vi "DiffDrivePoseEst2_UpdateWithTime.vi"(6 "CurrentTimeSeconds":dbl=-1.0, 8 "RightDistance":dbl, 9 "LeftDistance":dbl, 10 "GyroAngle":T3={"VALUE"=0.0, "COS"=1.0, "SIN"=0.0} {"SIN" format="%13.4f"; "COS" format="%13.4f"; "VALUE" format="%13.4f"}, 11 "in DiffDrivePoseEst2":T4={"M_Vision_K"=[], "m_nominal_dT"=0.0, "m_PrevTime_Sec"=0.0, "Pose_Buffer"={"TimeStamps"=[], "DataArray"=[], "Min_TimeStamp"=0.0, "Max_TimeStamp"=0.0, "ItemCount"=0, "MaxBufferTime"=0.0}, "Diff_Drive_Kinematics"={"TrackWidth_Meters"=0.0}, "Diff_Drive_Odom_2"={"M_POSE_Meters"={"TRANSLATION"={"X"=0.0, "Y"=0.0}, "ROTATION"={"VALUE"=0.0, "COS"=1.0, "SIN"=0.0}}, "M_GyroOffset"={"VALUE"=0.0, "COS"=1.0, "SIN"=0.0}, "M_PrevAngle"={"VALUE"=0.0, "COS"=1.0, "SIN"=0.0}, "M_PrevLeftDist_M"=0.0, "M_PrevRightDist_M"=0.0, "M_InitLeftDist_M"=0.0, "M_InitRightDist_M"=0.0}, "M_Q"=[[0.0], [0.0], [0.0]]} {"Diff_Drive_Odom_2"."M_PrevAngle"."SIN" format="%13.4f"; "Diff_Drive_Odom_2"."M_PrevAngle"."COS" format="%13.4f"; "Diff_Drive_Odom_2"."M_PrevAngle"."VALUE" format="%13.4f"; "Diff_Drive_Odom_2"."M_GyroOffset"."SIN" format="%13.4f"; "Diff_Drive_Odom_2"."M_GyroOffset"."COS" format="%13.4f"; "Diff_Drive_Odom_2"."M_GyroOffset"."VALUE" format="%13.4f"; "Diff_Drive_Odom_2"."M_POSE_Meters"."ROTATION"."SIN" format="%13.4f"; "Diff_Drive_Odom_2"."M_POSE_Meters"."ROTATION"."COS" format="%13.4f"; "Diff_Drive_Odom_2"."M_POSE_Meters"."ROTATION"."VALUE" format="%13.4f"; "Diff_Drive_Odom_2"."M_POSE_Meters"."TRANSLATION"."Y" format="%14.3f"; "Diff_Drive_Odom_2"."M_POSE_Meters"."TRANSLATION"."X" format="%14.3f"; "Diff_Drive_Kinematics"."TrackWidth_Meters" format="%20.4f"}) -> (0 "Error":bool, 2 "Estimated Pose":T1 {"ROTATION"."SIN" format="%13.4f"; "ROTATION"."COS" format="%13.4f"; "ROTATION"."VALUE" format="%13.4f"; "TRANSLATION"."Y" format="%14.3f"; "TRANSLATION"."X" format="%14.3f"}, 3 "Out DiffDrivePoseEst2":T4={"M_Vision_K"=[], "m_nominal_dT"=0.0, "m_PrevTime_Sec"=0.0, "Pose_Buffer"={"TimeStamps"=[], "DataArray"=[], "Min_TimeStamp"=0.0, "Max_TimeStamp"=0.0, "ItemCount"=0, "MaxBufferTime"=0.0}, "Diff_Drive_Kinematics"={"TrackWidth_Meters"=0.0}, "Diff_Drive_Odom_2"={"M_POSE_Meters"={"TRANSLATION"={"X"=0.0, "Y"=0.0}, "ROTATION"={"VALUE"=0.0, "COS"=1.0, "SIN"=0.0}}, "M_GyroOffset"={"VALUE"=0.0, "COS"=1.0, "SIN"=0.0}, "M_PrevAngle"={"VALUE"=0.0, "COS"=1.0, "SIN"=0.0}, "M_PrevLeftDist_M"=0.0, "M_PrevRightDist_M"=0.0, "M_InitLeftDist_M"=0.0, "M_InitRightDist_M"=0.0}, "M_Q"=[[0.0], [0.0], [0.0]]} {"Diff_Drive_Odom_2"."M_PrevAngle"."SIN" format="%13.4f"; "Diff_Drive_Odom_2"."M_PrevAngle"."COS" format="%13.4f"; "Diff_Drive_Odom_2"."M_PrevAngle"."VALUE" format="%13.4f"; "Diff_Drive_Odom_2"."M_GyroOffset"."SIN" format="%13.4f"; "Diff_Drive_Odom_2"."M_GyroOffset"."COS" format="%13.4f"; "Diff_Drive_Odom_2"."M_GyroOffset"."VALUE" format="%13.4f"; "Diff_Drive_Odom_2"."M_POSE_Meters"."ROTATION"."SIN" format="%13.4f"; "Diff_Drive_Odom_2"."M_POSE_Meters"."ROTATION"."COS" format="%13.4f"; "Diff_Drive_Odom_2"."M_POSE_Meters"."ROTATION"."VALUE" format="%13.4f"; "Diff_Drive_Odom_2"."M_POSE_Meters"."TRANSLATION"."Y" format="%14.3f"; "Diff_Drive_Odom_2"."M_POSE_Meters"."TRANSLATION"."X" format="%14.3f"; "Diff_Drive_Kinematics"."TrackWidth_Meters" format="%20.4f"})   [LabVIEW 2019, in "Trajectory_Library.lvlib"]
doc: "Updates the the Unscented Kalman Filter using only wheel encoder information. Note that this should be called every loop.\n\nInputs:\n - LeftSpeed -- Left wheel speed (meters/sec)\n - RightSpeed -- Right wheel speed (meters/sec)\n - inDiffDrivePoseEst -- system data cluster\n - gyroAngle -- The current gyro angle. (radians)\n - currentTime -- Time at which this method was called, in seconds.\n - distanceLeftMeters -- The total distance travelled by the left wheel in meters. This can be the encoder reading.\n - distanceRightMeters -- The total distance travelled by the right wheel in meters. This can be the encoder reading.\n\nOutputs:\n - outDiffDrivePoseEst -- system data cluster\n - EstimatedPose -- The estimated pose of the robot in meters."
uses:
  Trajectory_Library.lvlib
  <vilib>/Analysis/Matrix/Datatypes/RealMatrix.ctl
  <vilib>/Analysis/Matrix/NI_Matrix.lvlib
  TypeDef/ROTATION2D.ctl
  TypeDef/TRANSLATION2D.ctl
  TypeDef/POSE2D.ctl
  TypeDef/TIME_INTERPOLATABLE_VARIANT.ctl
  TypeDef/DIFF_DRIVE_KINEMATICS.ctl
  TypeDef/DIFF_DRIVE_ODOM2.ctl
  TypeDef/DIFF_DRIVE_POSE_EST2.ctl
panel:
  # "<3, 1>"
  # "<3, 3>"
  # "<3, 1>"
  # "<3, 3>"
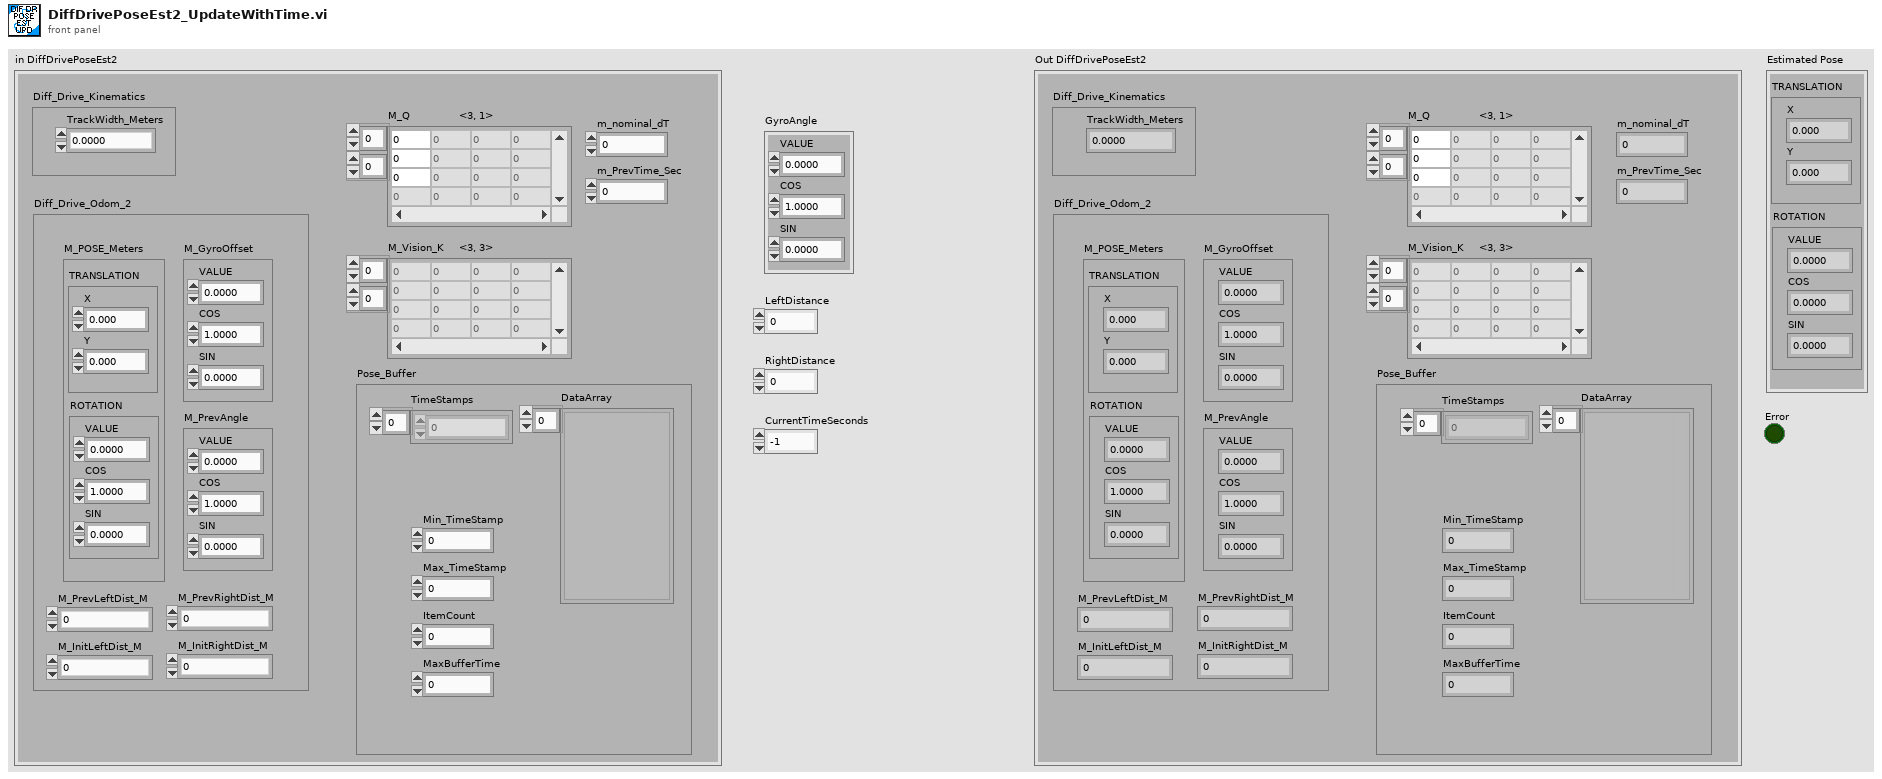
[diagram p1: front panel]
types:
  T1 = typedef "Trajectory_Library.lvlib/POSE2D.ctl" = cluster{"TRANSLATION":T2, "ROTATION":T3}
  T2 = typedef "Trajectory_Library.lvlib/TRANSLATION2D.ctl" = cluster{"X":dbl, "Y":dbl}
  T3 = typedef "Trajectory_Library.lvlib/ROTATION2D.ctl" = cluster{"VALUE":dbl, "COS":dbl, "SIN":dbl}
  T4 = typedef "Trajectory_Library.lvlib/DIFF_DRIVE_POSE_EST2.ctl" = cluster{"M_Vision_K":T5, "m_nominal_dT":dbl, "m_PrevTime_Sec":dbl, "Pose_Buffer":T6, "Diff_Drive_Kinematics":T7, "Diff_Drive_Odom_2":T8, "M_Q":T5}
  T5 = typedef "NI_Matrix.lvlib/RealMatrix.ctl" = dbl[][]
  T6 = typedef "Trajectory_Library.lvlib/TIME_INTERPOLATABLE_VARIANT.ctl" = cluster{"TimeStamps":dbl[], "DataArray":variant[], "Min_TimeStamp":dbl, "Max_TimeStamp":dbl, "ItemCount":i32, "MaxBufferTime":dbl}
  T7 = typedef "Trajectory_Library.lvlib/DIFF_DRIVE_KINEMATICS.ctl" = cluster{"TrackWidth_Meters":dbl}
  T8 = typedef "Trajectory_Library.lvlib/DIFF_DRIVE_ODOM2.ctl" = cluster{"M_POSE_Meters":T1, "M_GyroOffset":T3, "M_PrevAngle":T3, "M_PrevLeftDist_M":dbl, "M_PrevRightDist_M":dbl, "M_InitLeftDist_M":dbl, "M_InitRightDist_M":dbl}
  T9 = typedef "Trajectory_Library.lvlib/DIFF_DRIVE_POSE_EST2_INTERP_RECORD.ctl" = cluster{"PoseMeters":T1, "GyroAngle":T3, "LeftMeters":dbl, "RightMeters":dbl}
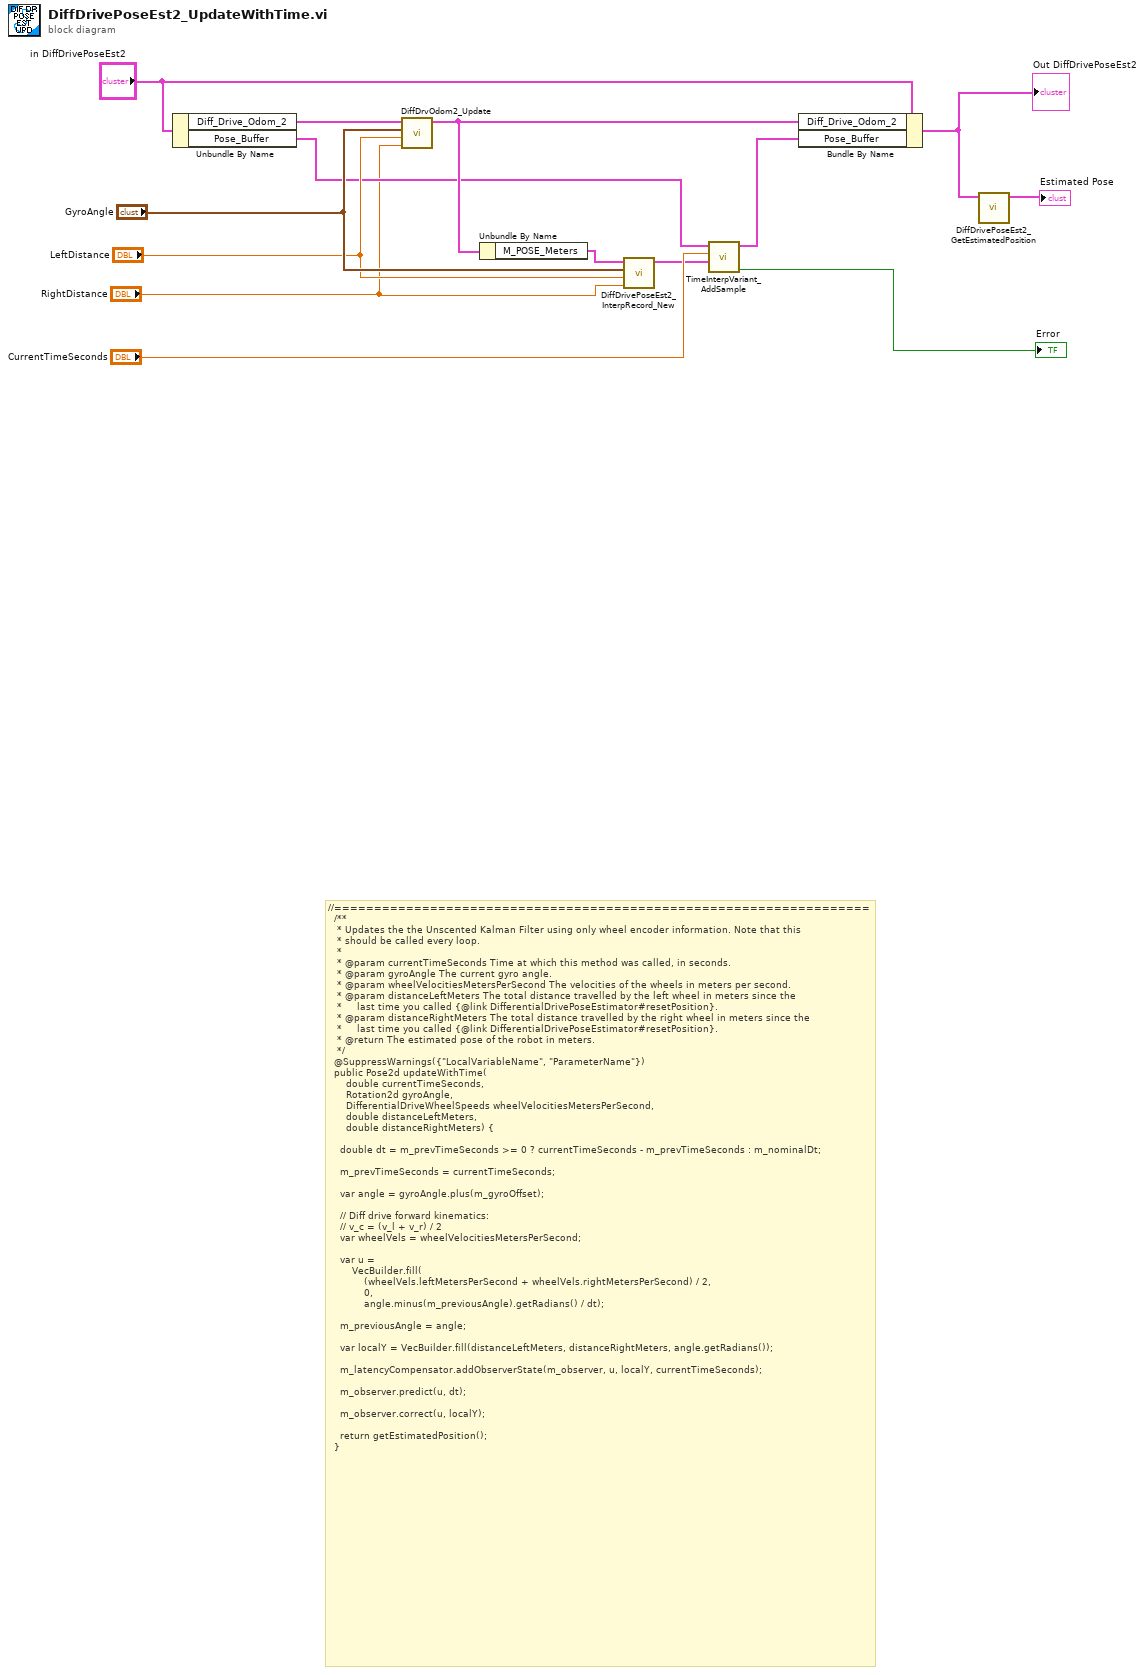
[diagram p0: block diagram]
diagram:
  # "//===================================================================\n  /**\n   * Updates the the Unscented Kalman Filter using only wheel encoder information. Note that this\n   * should be called every loop.\n   *\n   * @param currentTimeSeconds Time at which this method was called, in seconds.\n   * @param gyroAngle The current gyro angle.\n   * @param wheelVelocitiesMetersPerSecond The velocities of the wheels in meters per second.\n   * @param distanceLeftMeters The total distance travelled by the left wheel in meters since the\n   *     last time you called {@link DifferentialDrivePoseEstimator#resetPosition}.\n   * @param distanceRightMeters The total distance travelled by the right wheel in meters since the\n   *     last time you called {@link DifferentialDrivePoseEstimator#resetPosition}.\n   * @return The estimated pose of the robot in meters.\n   */\n  @SuppressWarnings({\"LocalVariableName\", \"ParameterName\"})\n  public Pose2d updateWithTime(\n      double currentTimeSeconds,\n      Rotation2d gyroAngle,\n      DifferentialDriveWheelSpeeds wheelVelocitiesMetersPerSecond,\n      double distanceLeftMeters,\n      double distanceRightMeters) {\n\n    double dt = m_prevTimeSeconds >= 0 ? currentTimeSeconds - m_prevTimeSeconds : m_nominalDt;\n\n    m_prevTimeSeconds = currentTimeSeconds;\n\n    var angle = gyroAngle.plus(m_gyroOffset);\n\n    // Diff drive forward kinematics:\n    // v_c = (v_l + v_r) / 2\n    var wheelVels = wheelVelocitiesMetersPerSecond;\n\n    var u =\n        VecBuilder.fill(\n            (wheelVels.leftMetersPerSecond + wheelVels.rightMetersPerSecond) / 2,\n            0,\n            angle.minus(m_previousAngle).getRadians() / dt);\n\n    m_previousAngle = angle;\n\n    var localY = VecBuilder.fill(distanceLeftMeters, distanceRightMeters, angle.getRadians());\n\n    m_latencyCompensator.addObserverState(m_observer, u, localY, currentTimeSeconds);\n\n    m_observer.predict(u, dt);\n\n    m_observer.correct(u, localY);\n\n    return getEstimatedPosition();\n  }"
  n1 = Unbundle By Name("in DiffDrivePoseEst2") -> ("Diff_Drive_Odom_2"=w14:T8, "Pose_Buffer"=w8:T6)
  n2 = call "DiffDrvOdom2_Update.vi"("Right Distance M"="RightDistance", "Left Distance M"="LeftDistance", "Gyro Reading"="GyroAngle", "In DIFF_DRIVE_ODOM"=w14) -> ("Out DIFF_DRIVE_ODOM"=w12:T8)  [unwired: 6 in, 1 out]
  n3 = Unbundle By Name(w12) -> ("M_POSE_Meters"=w11:T1)
  n4 = call "DiffDrivePoseEst2_InterpRecord_New.vi"("RightDistance"="RightDistance", "LeftDistance"="LeftDistance", "GyroAngle"="GyroAngle", "M_POSE_Meters"=w11) -> ("DIFF_DRIVE_POSE_EST2_INTERP_RECORD"=w6:T9)  [unwired: 7 in]
  n5 = call "TimeInterpVariant_AddSample.vi"("Variant"=w6, "TimeStamp"="CurrentTimeSeconds", "in TimeInterpVariant"=w8) -> ("Error"=→"Error":bool, "out TimeInterpVariant"=w5:T6)  [unwired: 7 in]
  n6 = Bundle By Name(cluster="in DiffDrivePoseEst2", "Diff_Drive_Odom_2"=w12, "Pose_Buffer"=w5) -> (w3:T4)
  "Out DiffDrivePoseEst2" <- w3
  n7 = call "DiffDrivePoseEst2_GetEstimatedPosition.vi"("in DiffDrivePoseEstimate"=w3) -> ("Estimated Pose"=→"Estimated Pose":T1)  [unwired: 10 in]
